vi "Lockin - exponential.vi"(8 "X array (min)":dbl[](array[numeric]), 9 "Tx (min)":dbl, 10 "phase":dbl, 11 "A":dbl) -> (0 "Y array OUT":cdb[](array[numeric]))   [LabVIEW 2012]
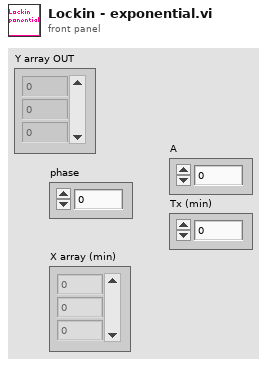
[diagram p1: front panel]
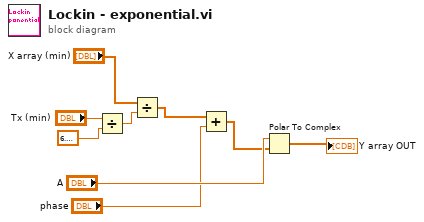
[diagram p0: block diagram]
diagram:
  n1 = Divide(x="Tx (min)", y=6.283185307179586) -> (x/y=w6:dbl)
  n2 = Divide(x="X array (min)", y=w6) -> (x/y=w3:dbl[])
  n3 = Add(x=w3, y="phase") -> (x+y=w2:dbl[])
  n4 = Polar To Complex(1:w2, 2:"A") -> (0:→"Y array OUT":cdb[])
